vi "sub_AO_main.vi"(8 "error in":errorcluster) -> (0 "error out":errorcluster)   [LabVIEW 2019]
uses:
  _ctrl/create-rw-close.ctl
  _ctrl/init-w-close.ctl
  SubVIs/common/Glob_Ref.vi
panel:
  out "n":i32
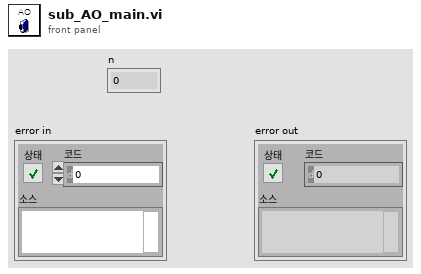
[diagram p1: front panel]
types:
  T1 = typedef "create-rw-close.ctl" = enum16{"create", "write", "read", "delete", "close"}
  T2 = typedef "init-w-close.ctl" = enum16{"open", "init", "write", "close"}
  T3 = typedef "AO_q-data.ctl" = enum16{"init", "AO start"}
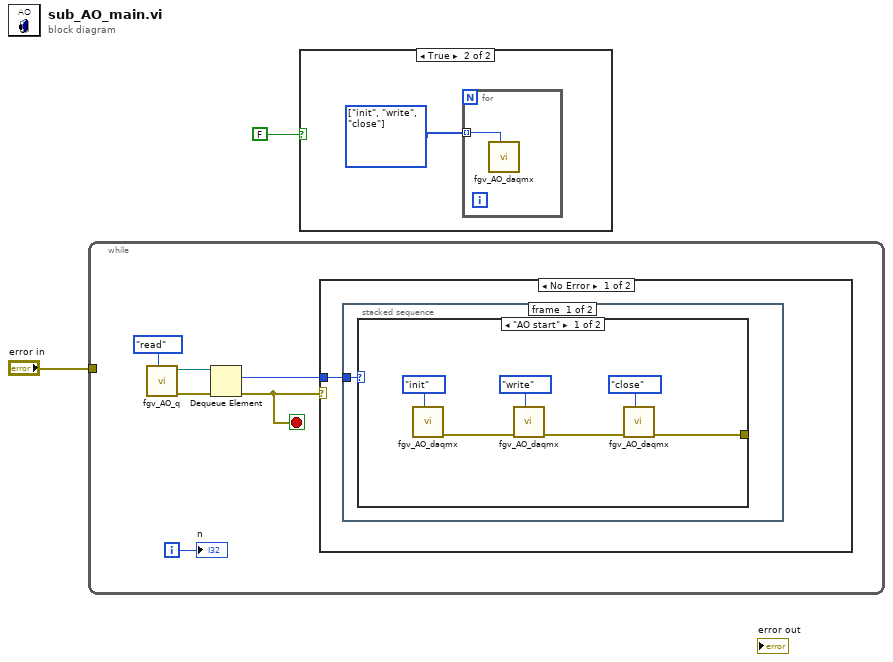
[diagram p0: block diagram]
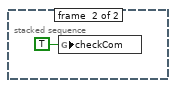
[diagram p4: hidden frame]
diagram:
  n1 = while {
    tunnel: "error in" -> [_]
    i -> [w3]
    stop <- w4 stop-if-true
    n2 = call "fgv_AO_q.vi"("cmd"=create-rw-close."read") -> ("error out"=w6:errorcluster, "queue out"=w7:refnum<queue>)  [unwired: 9 in]
    n3 = Dequeue Element(queue=w7, error in (no error)=w6) -> (element=w5:T3, error out=w4:errorcluster)  [unwired: 1 in, 2 out]
    n4 = case shown="No Error" w4 {
      tunnel: w5 -> [w9 _]
      frame No Error {
        n5 = stacked-sequence {
          tunnel: w9 -> [w10 _]
          frame #0 {
            n6 = case shown="\"AO start\"" w10 {
              tunnel: [w11 _] -> _
              frame "AO start" {
                n7 = call "fgv_AO_daqmx.vi"("cmd"=init-w-close."init") -> ("error out"=w13:errorcluster)  [unwired: 10 in]
                n8 = call "fgv_AO_daqmx.vi"("cmd"=init-w-close."write", "error in"=w13) -> ("error out"=w12:errorcluster)  [unwired: 9 in]
                n9 = call "fgv_AO_daqmx.vi"("cmd"=init-w-close."close", "error in"=w12) -> ("error out"=w11:errorcluster)  [unwired: 9 in]
              }
              frame "init", Default {
              }
            }
          }
          frame #1 {
            n10 = global write "Glob_Ref.vi" "checkCom"(TRUE ("checkCom")) -> ()
          }
        }
      }
      frame Error {
      }
    }
    "n" <- w3
  }
  n11 = case shown="True" FALSE {
    frame False {
    }
    frame True {
      w18 = T2[] [enum."init", enum."write", enum."close"] items=["open", "init", "write", "close"]
      n12 = for {
        tunnel: w18 -> [w19] mode=indexing
        n13 = call "fgv_AO_daqmx.vi"("cmd"=w19) -> ()  [unwired: 10 in, 1 out]
      }
    }
  }
